vi "Write to Temp File.vi"(6 "Append to file?":bool, 7 "Single Channel?":bool, 8 "error in (no error)":errorcluster, 9 "Dev2 Zero Values":dbl[](array[numeric]), 10 "Dev1 Zero Values":dbl[](array[numeric]), 11 "Waveform Array":waveform(dbl)[][](array[waveform])) -> (0 "error out":errorcluster, 2 "Force Outputs":dbl[](array[numeric]), 3 "Zeroed Array":waveform(dbl)[][](array[waveform]))   [LabVIEW 2017]
uses:
  <vilib>/Waveform/WDTFileIO.llb/ Write Waveforms to File (1D).vi
panel:
  out "Dev2_Fx":dbl
  out "Dev2_Fy":dbl
  out "Dev2_Fy":dbl
  out "Dev1_Fx":dbl
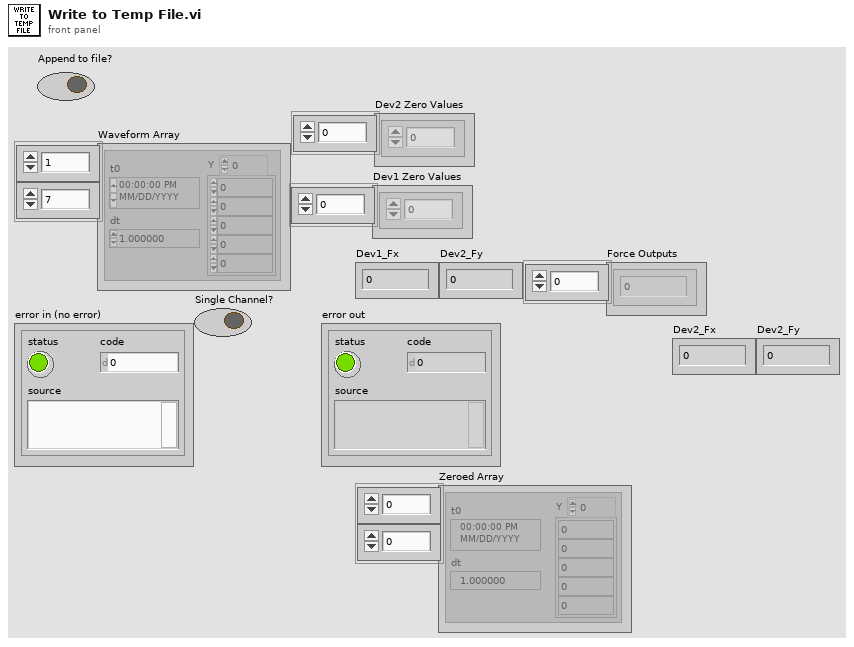
[diagram p1: front panel]
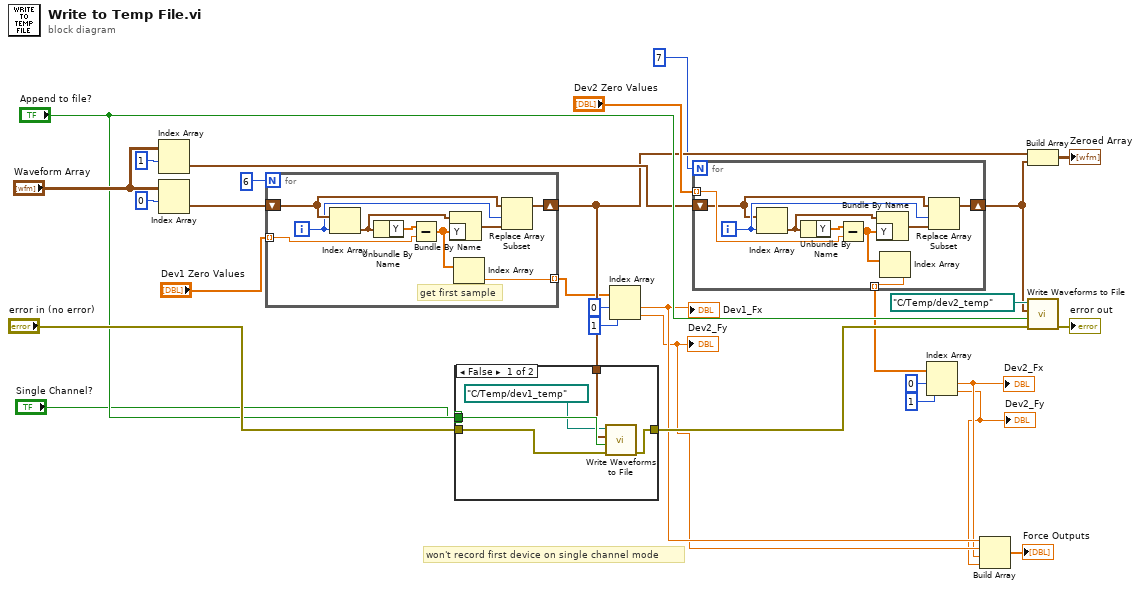
[diagram p0: block diagram]
diagram:
  # "won't record first device on single channel mode"
  n1 = Index Array(array="Waveform Array", index (row)=1) -> (element=w22:waveform(dbl)[])  [unwired: 1 in]
  n2 = Index Array(array="Waveform Array", index (row)=0) -> (element=w14:waveform(dbl)[])  [unwired: 1 in]
  n3 = for {
    N: 6 -> [_]
    tunnel: "Dev1 Zero Values" -> [w37] mode=indexing
    shift-right: [w32] -> w21
    shift-left: w14 -> [w35]
    tunnel: [w30] -> w11 mode=indexing
    i -> [w34]
    # "get first sample"
    n4 = Index Array(array=w35, index=w34) -> (element=w36:waveform(dbl))
    n5 = Unbundle By Name(w36) -> ("Y"=w38:dbl[])
    n6 = Subtract(x=w38, y=w37) -> (x-y=w31:dbl[])
    n7 = Bundle By Name(cluster=w36, "Y"=w31) -> (w33:waveform(dbl))
    n8 = Index Array(array=w31) -> (element=w30:dbl)  [unwired: 1 in]
    n9 = Replace Array Subset(array=w35, new element=w33, index=w34) -> (w32:waveform(dbl)[])
  }
  n10 = case shown="False" "Single Channel?" {
    tunnel: "error in (no error)" -> [w43 w44]
    tunnel: "Append to file?" -> [w42 _]
    tunnel: [w41 w44] -> w25
    tunnel: w21 -> [w40 _]
    frame False {
      n11 = call-poly <vilib>:"Write Waveforms to File.vi"("error in (no error)"=w43, "append to file? (new file:F)"=w42, "waveform array"=w40, "file path (dialog if empty)"=path "C:/Temp/dev1_temp") -> ("error out"=w41:errorcluster)  [unwired: 6 in, 1 out]
    }
    frame True {
    }
  }
  n12 = Index Array(array=w11, index #1=0 ("index"), index #2=1 ("index")) -> (element #1=w5:dbl, element #2=w4:dbl)
  "Dev1_Fx" <- w5
  "Dev2_Fy" <- w4
  n13 = for {
    N: 7 -> [_]
    tunnel: "Dev2 Zero Values" -> [w52] mode=indexing
    shift-right: [w47] -> w18
    shift-left: w22 -> [w49]
    tunnel: [w45] -> w6 mode=indexing
    i -> [w50]
    n14 = Index Array(array=w49, index=w50) -> (element=w51:waveform(dbl))
    n15 = Unbundle By Name(w51) -> ("Y"=w53:dbl[])
    n16 = Subtract(x=w53, y=w52) -> (x-y=w46:dbl[])
    n17 = Bundle By Name(cluster=w51, "Y"=w46) -> (w48:waveform(dbl))
    n18 = Index Array(array=w46) -> (element=w45:dbl)  [unwired: 1 in]
    n19 = Replace Array Subset(array=w49, new element=w48, index=w50) -> (w47:waveform(dbl)[])
  }
  n20 = Index Array(array=w6, index #1=0 ("index"), index #2=1 ("index")) -> (element #1=w3:dbl, element #2=w2:dbl)
  "Dev2_Fx" <- w3
  "Dev2_Fy" <- w2
  n21 = Build Array(w5, w4, w3, w2) -> (→"Force Outputs":dbl[])
  n22 = Build Array(w21, w18) -> (→"Zeroed Array":waveform(dbl)[][])
  n23 = call-poly <vilib>:"Write Waveforms to File.vi"("error in (no error)"=w25, "append to file? (new file:F)"="Append to file?", "waveform array"=w18, "file path (dialog if empty)"=path "C:/Temp/dev2_temp") -> ("error out"=→"error out":errorcluster)  [unwired: 6 in, 1 out]
